vi "Set DS Alert Text.vi"(8 "error in (no error)":errorcluster, 11 "handle":i64) -> (0 "error out":errorcluster)   [LabVIEW 2026, in "MrcLib.lvlib"]
doc: "Update the text for the referenced Alert"
uses:
  MrcLib.lvlib
panel:
  in  "text":string
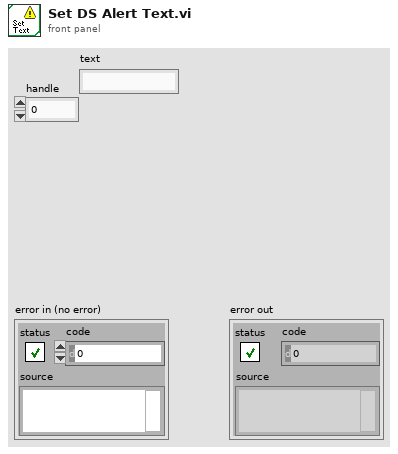
[diagram p1: front panel]
types:
  T1 = typedef "MRC String.ctl" = cluster{"pointer":u64, "length":u64}
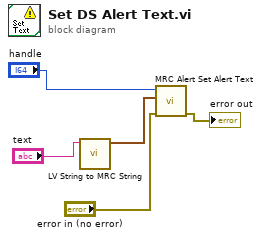
[diagram p0: block diagram]
diagram:
  n1 = call "LV String to MRC String.vi"("LV String"="text") -> ("MRC String"=w4:T1)  [unwired: 10 in]
  n2 = call "MRC Alert Set Alert Text.vi"("error in (no error)"="error in (no error)", "text"=w4, "handle"="handle") -> ("error out"=→"error out":errorcluster)  [unwired: 8 in]
